vi "initializeSMC.vi"(8 "error in (no error)":errorcluster, 10 "Controller address":i32=1, 11 "VisaRresourceName":string="VisaResourceName") -> (3 "Device Connection Cluster":T1)   [LabVIEW 2020]
panel:
  out "GPIB? ( T - GPIB, F - RS232 )":bool
  out "error (duplicate)":errorcluster
  out "VISA resource name (duplicate)":refnum<visa-resource-name>
  in  "XON/XOFF (False)":bool
  in  "Baud Rate (921600 - USB)":u32=57600 min=300 max=115200 step=300
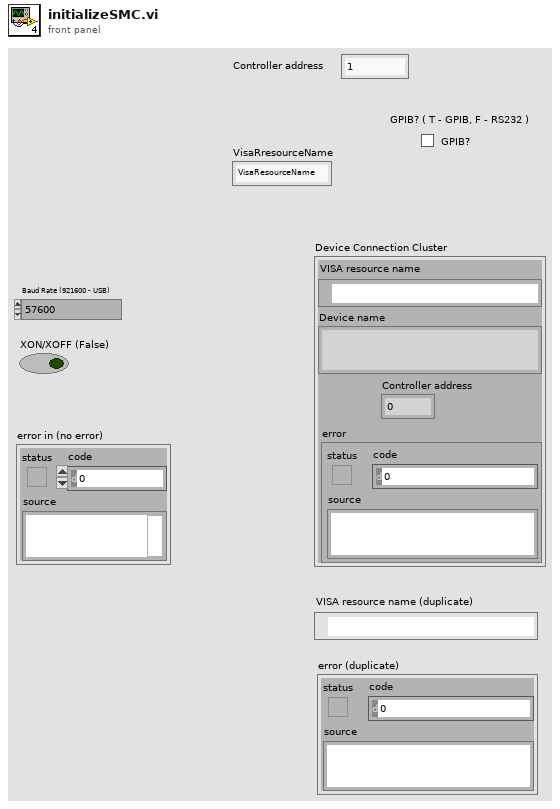
[diagram p1: front panel]
types:
  T1 = cluster{"VISA resource name":refnum<visa-resource-name>, "Device name":string, "Controller address":i32, "error":errorcluster}
  T2 = cluster{"VISA resource name":refnum<visa-resource-name>, "search string/char (-)":string, "Controller address":i32, "error out":errorcluster}
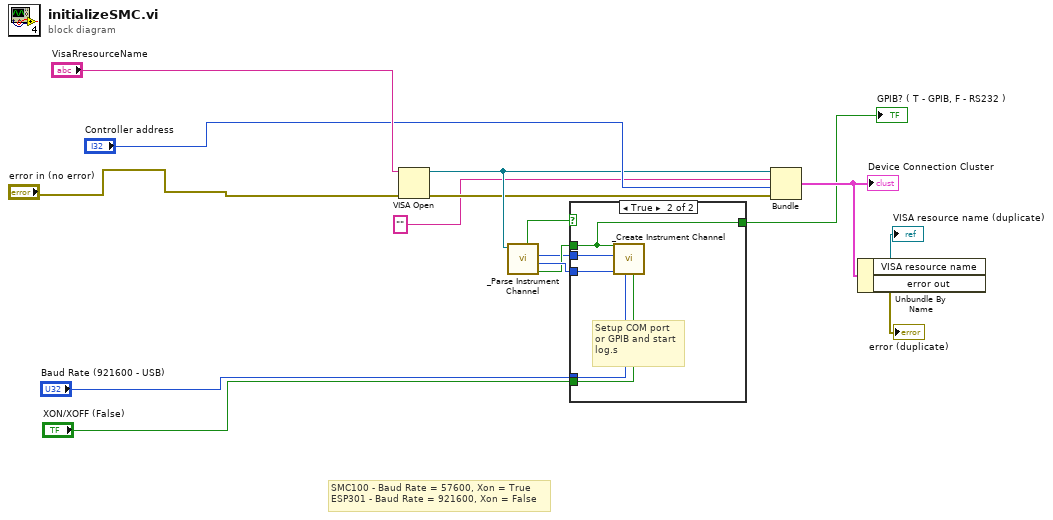
[diagram p0: block diagram]
diagram:
  # "SMC100 - Baud Rate = 57600, Xon = True\nESP301 - Baud Rate = 921600, Xon = False"
  n1 = VISA Open(error in (no error)="error in (no error)", VISA resource name="VisaRresourceName") -> (VISA resource name=w8:refnum<visa-resource-name>, error out=w7:errorcluster)  [unwired: 3 in]
  n2 = call "_Parse Instrument Channel.vi"("Instrument Channel"=w8) -> ("T - GPIB, F - RS232"=w3:bool, "Hardware Address"=w4:i32, "Instrument Address"=w2:i16, "Valid String"=w1:bool)  [unwired: 6 in, 1 out]
  n3 = case shown="True" w1 {
    selector: w1 -> [w17 _]
    tunnel: w4 -> [_ w22]
    tunnel: w3 -> [_ w19]
    tunnel: w2 -> [_ w21]
    tunnel: "Baud Rate (921600 - USB)" -> [_ w20]
    tunnel: [w17 w19] -> w11
    tunnel: "XON/XOFF (False)" -> [_ w18]
    frame False {
    }
    frame True {
      # "Setup COM port\nor GPIB and start\nlog.s"
      n4 = call "_Create Instrument Channel.vi"("XON/XOFF (False)"=w18, "Baud Rate (921600 - USB)"=w20, "COM Port (1)"=w22, "GPIB Primary Address (4)"=w21, "(F), T - GPIB, F - RS232"=w19) -> ()  [unwired: 4 in, 3 out]
    }
  }
  "GPIB? ( T - GPIB, F - RS232 )" <- w11
  n5 = Bundle("VISA resource name"=w8, "search string/char (-)"="", "Controller address"="Controller address", "error out"=w7) -> (w14:T2)  [unwired: 1 in]
  "Device Connection Cluster" <- w14
  n6 = Unbundle By Name(w14) -> ("VISA resource name"=→"VISA resource name (duplicate)":refnum<visa-resource-name>, "error out"=→"error (duplicate)":errorcluster)
